vi "Init Refs.vi"(10 "Refs":T1) -> (2 "Refs":refnum<class "Refs.lvclass">)   [LabVIEW 2025, in "_Template.lvlib" / "Templates.lvlib" / "TEMPLATE Actor.lvlib" / "TEMPLATE Actor.lvlib" / "TEMPLATE Refs.lvlib"]
uses:
  TEMPLATE Refs.lvlib
  jettl/jettl/Refs/Refs.lvclass
  Refs.ctl
  TEMPLATE Refs/TEMPLATE Refs.lvclass
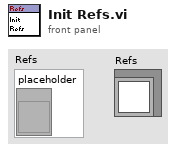
[diagram p1: front panel]
types:
  T1 = typedef "_Template.lvlib/Templates.lvlib/TEMPLATE Actor.lvlib/TEMPLATE Actor.lvlib/TEMPLATE Refs.lvlib/Refs.ctl" = cluster{"placeholder":refnum<vi>}
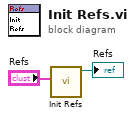
[diagram p0: block diagram]
diagram:
  n1 = call "Init Refs.vi"("Refs"="Refs") -> ("TEMPLATE Refs out"=→"Refs":refnum<class "TEMPLATE Refs.lvclass">)  [unwired: 10 in]
